vi "GUIAS CURVAS EM FUNÇÃO DO RAIO-3.vi"() -> ()   [LabVIEW 2014]
uses:
  <vilib>/Platform/TimedLoop/XDataNode/timing_clust.ctl
  <vilib>/Platform/TimedLoop/XDataNode/nitl_modes.ctl
  <vilib>/Platform/TimedLoop/XDataNode/wakeup.ctl
  <vilib>/Platform/TimedLoop/XDataNode/XDataNode.xnode
  <userlib>/Newport ESP301/Newport ESP301.lvlib
  <vilib>/Platform/TimedLoop/XDataNode/XDNodeRunTimeDep.lvlib
  <vilib>/Instr/_visa.llb/VISA Configure Serial Port (Instr).vi
panel:
  out "Raio":dbl
  out "PROGRESSÃO":i32
  in  "Raios":dbl[](array[numeric])=[100.0]
  in  "N_Guias":dbl=1.0
  in  "Iniciar":bool
  out "sin(x)":dbl
  in  "L":dbl=10.0 format="%.1f"
  in  "In.Curva":dbl=2.0
  out "Yin":dbl format="%.6g"
  out "Xin":dbl format="%.6g"
  out "d (um)":dbl
  in  "dist.":dbl=100.0
  in  "Stop Button":bool
  out "error out":errorcluster
  out "X (mm)":dbl format="%.2g"
  out "Y (um)":dbl format="%.1f"
  out "XY Graph":cluster{dbl[], dbl[]}(graph)={[0.0, 0.0, 0.0, 0.0, 0.0, 0.0, 0.0, 0.0, 0.0, 0.0, 0.0, 0.0, 0.0, 0.0, 0.0, 0.0, 0.0, 0.0, 0.0, 0.0, 0.0, 0.0, 0.0, 0.0, 0.0, 0.0, 0.0, 0.0, 0.0, 0.0, 0.0, 0.0, 0.0, 0.0, 0.0, 0.0, 0.0, 0.0, 0.0, 0.0, 0.0, 0.0, 0.0, 0.0, 0.0, 0.0, 0.0, 0.0, 0.0, 0.0, 0.0, 0.0, 0.0, 0.0, 0.0, 0.0, 0.0, 0.0, 0.0, 0.0, 0.0, 0.0, 0.0, 0.0, 0.0, 0.0, 0.0, 0.0, 0.0, 0.0, 0.0, 0.0, 0.0, 0.0, 0.0, 0.0], [4600.0, 4600.0, 4600.0, 4600.0, 4600.0, 4600.0, 4600.0, 4600.0, 4600.0, 4600.0, 4600.0, 4600.0, 4600.0, 4600.0, 4600.0, 4600.0, 4600.0, 4600.0, 4600.0, 4600.0, 4600.0, 4600.0, 4600.0, 4600.0, 4600.0, 4600.0, 4600.0, 4690.0, 4802.5, 4800.5, 4799.5, 4799.5, 4799.5, 4800.0, 4800.0, 4800.0, 4800.0, 4800.0, 4800.0, 4800.0, 4800.0, 4800.0, 4800.0, 4800.0, 4995.5, 5001.5, 5000.5, 5000.0, 5000.0, 4999.5, 4999.5, 5000.0, 5000.0, 5000.0, 5000.0, 5000.0, 5000.0, 5000.0, 5000.0, 5000.0, 5000.0, 5000.0, 5000.0, 5000.0, 5000.0, 5000.0, 5000.0, 5000.0, 5000.0, 5000.0, 5000.0, 5000.0, 5000.0, 5000.0, 5000.0, 5000.0]}
  in  "Refresh Button":bool
  in  "Velocity":dbl=3.0
  # "Inicio curva"
  # "Tamanho da amostra (mm)"
  # "Número guias curvas"
  # "Raio (mm)"
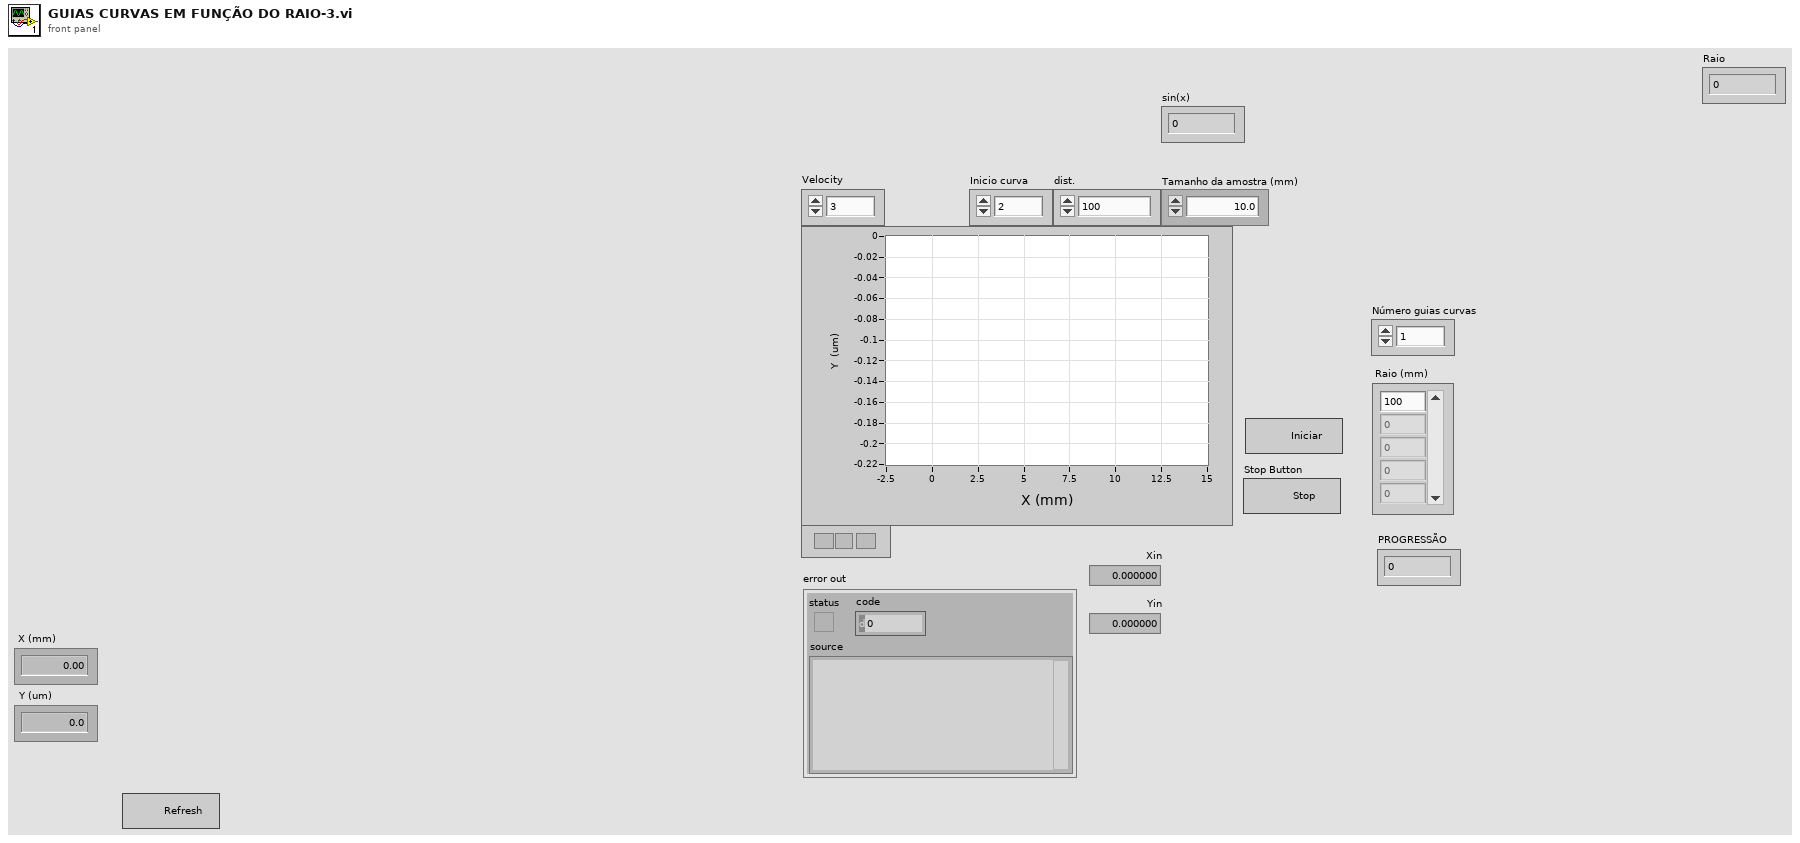
[diagram p1: front panel]
types:
  T1 = typedef "XDNodeRunTimeDep.lvlib/timing_clust.ctl" = cluster{"Expected End [f-1]":u64, "Actual End [f-1]":u64, "Finished Late? [f-1]":bool, "Expected End [i-1]":u64, "Actual End [i-1]":u64, "Finished Late? [i-1]":bool, "Expected Start [i]":u64, "Actual Start [i]":u64, "Expected Start [f]":u64, "Actual Start [f]":u64, "Source Name":string, "Structure Name":string, "Period":i64, "Deadline":i64, "Offset":i64, "Start":i64, "Priority":i32, "Timeout":i32, "Mode":T2, "Wakeup Reason":T3, "Error":errorcluster, "Source Type":string, "Secondary Source Type":string, "Global End Time":u64, "Global Start Time":u64, "Frame Duration":u64, "Iteration Duration":u64, "Assigned CPU":i32, "I/O Scan Engine Mode":u32}
  T2 = typedef "XDNodeRunTimeDep.lvlib/nitl_modes.ctl" = enum32{"No Change", "Process missed periods, maintain original phase", "Discard missed periods, maintain original phase", "Process missed periods, ignore original phase", "Discard missed periods, ignore original phase"}
  T3 = typedef "XDNodeRunTimeDep.lvlib/wakeup.ctl" = enum32{"Normal", "Aborted", "Asynchronous wakeup", "Timing source error", "Timed loop error", "Timeout"}
  T4 = cluster{"Axis1 moving":bool, "Axis2 moving":bool, "Axis3 moving":bool, "Axis4 moving":bool, "Motor Power of at least one axis":bool, "Reserved":bool, "Reserved":bool, "Reserved":bool, "Axis5 moving 2":bool, "Axis6 moving 2":bool, "Reserved":bool, "Reserved":bool, "Motor Power of at least one axis":bool, "Reserved":bool, "Reserved":bool, "Reserved":bool}
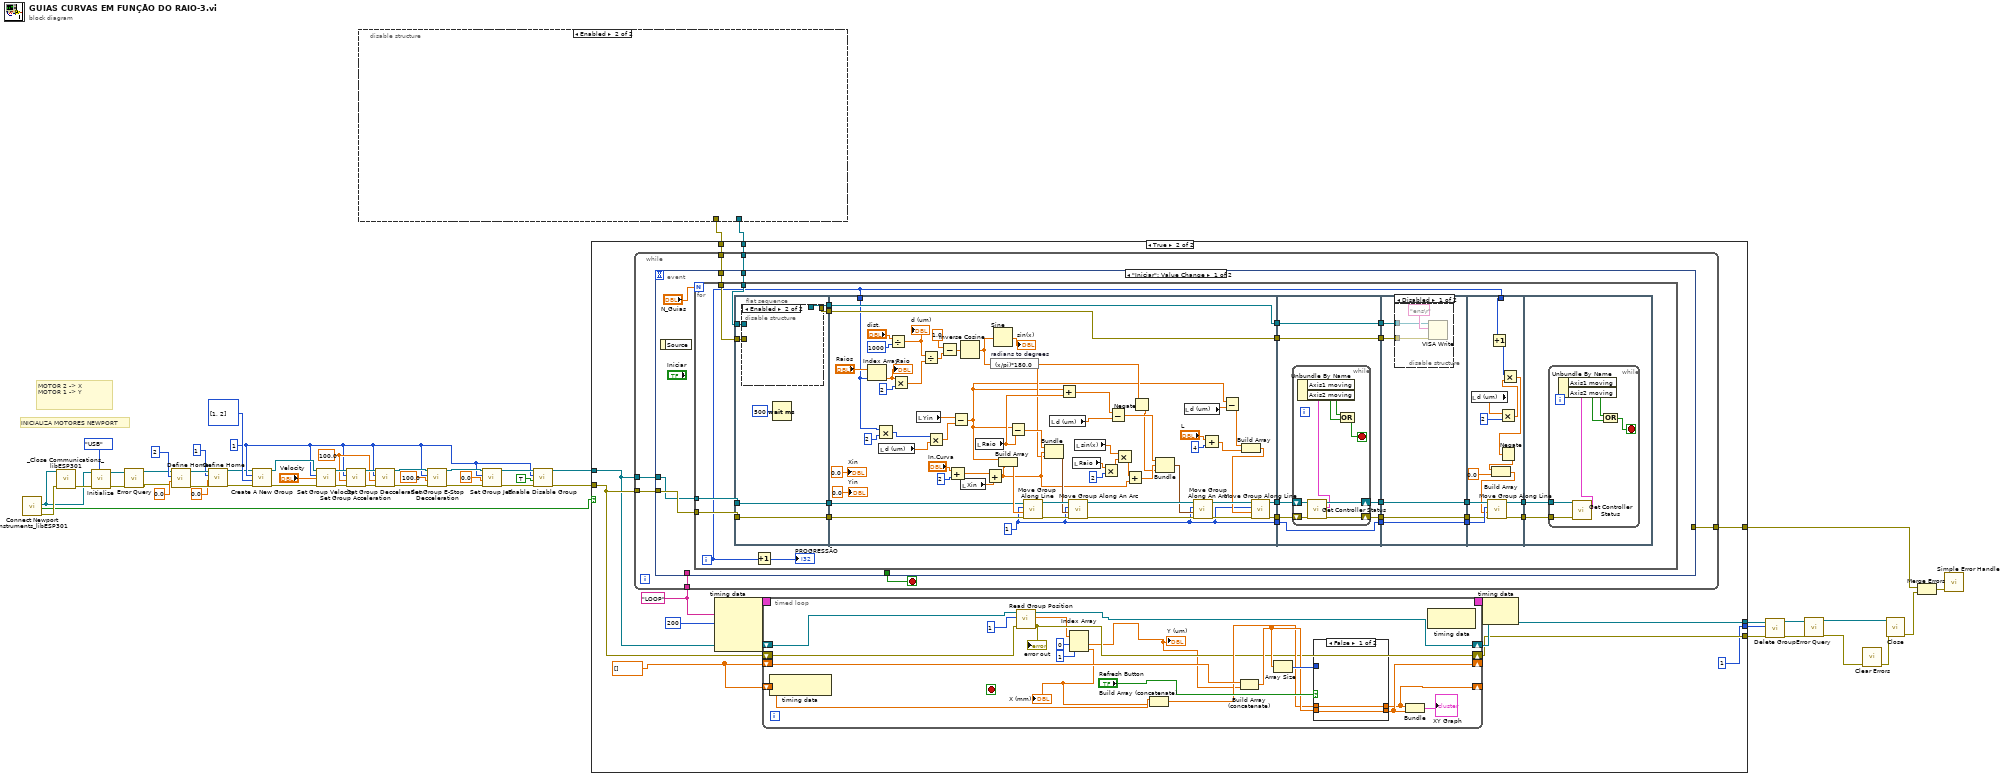
[diagram p0: block diagram]
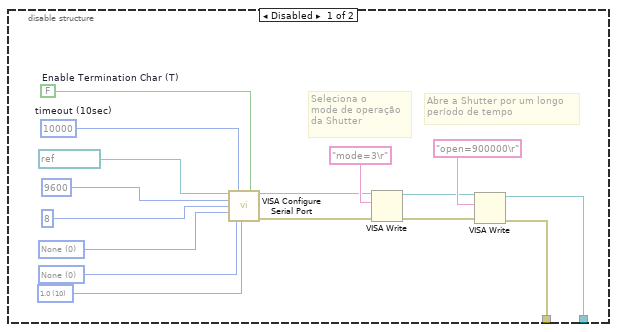
[diagram p2: hidden frame]
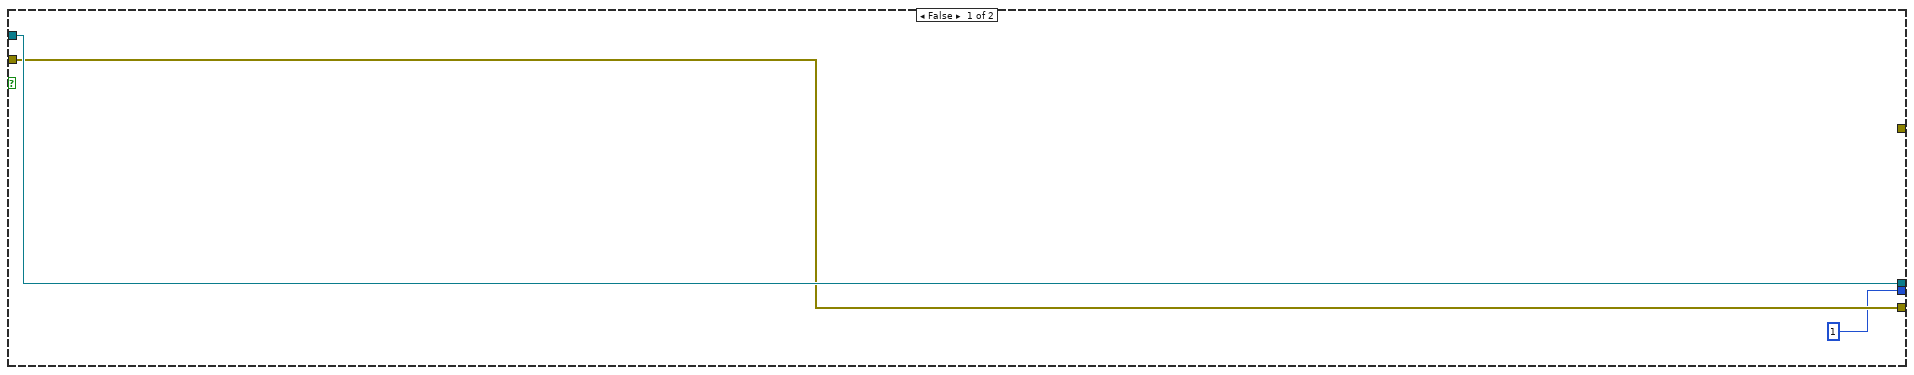
[diagram p3: hidden frame]
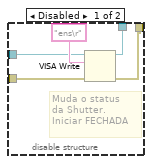
[diagram p4: hidden frame]
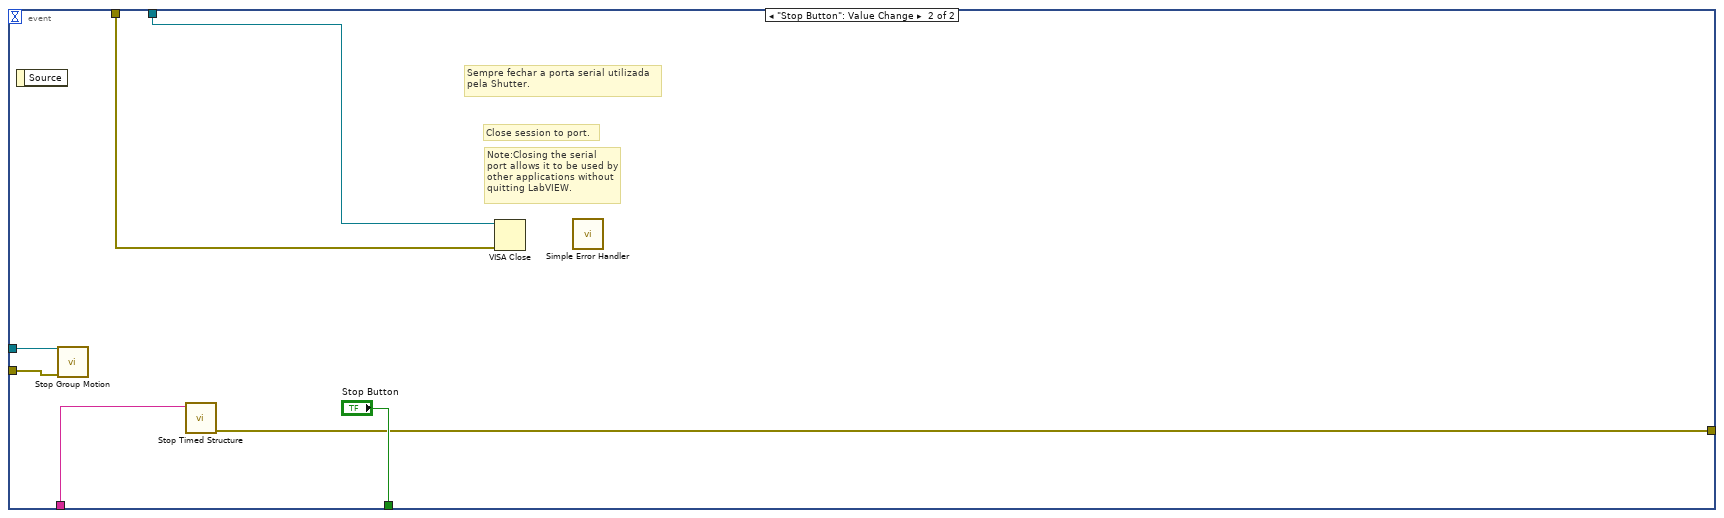
[diagram p6: hidden frame]
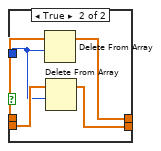
[diagram p7: hidden frame]
diagram:
  w21 = 1 ("Group #")
  w39 = 100.0 ("Acceleration (0 units/s²)")
  # "MOTOR 2 -> X\nMOTOR 1 -> Y"
  # "INICIALIZA MOTORES NEWPORT"
  n1 = call <userlib>:"Connect Newport Instruments_libESP301.vi"() -> ("error (duplicate)"=w49:errorcluster, "Connected"=w12:bool, "VISA resource name (duplicate)"=w48:refnum<visa-resource-name>)  [unwired: 7 in, 2 out]
  n2 = call <userlib>:"_Close Communications_libESP301.vi"("Instrument Channel"=w48, "error in (no error)"=w49) -> ("error out"=w51:errorcluster)  [unwired: 13 in]
  n3 = call <userlib>:"Initialize.vi"("VISA resource name"=w48, "error in (no error)"=w51, "Serial Link (RS232)"=enum16{"RS232", "USB"}."USB") -> ("VISA resource name out"=w29:refnum<visa-resource-name>, "error out"=w28:errorcluster)  [unwired: 6 in]
  n4 = call <userlib>:"Error Query.vi"("error in (no error)"=w28, "VISA resource name"=w29) -> ("error out"=w3:errorcluster, "VISA resource name out"=w4:refnum<visa-resource-name>)  [unwired: 2 in, 2 out]
  n5 = call <userlib>:"Define Home.vi"("error in (no error)"=w3, "Home Position (0 units)"=0.0, "Axis (1)"=2 ("y"), "VISA resource name"=w4) -> ("error out"=w9:errorcluster, "VISA resource name out"=w10:refnum<visa-resource-name>)  [unwired: 2 in]
  n6 = call <userlib>:"Define Home.vi"("error in (no error)"=w9, "Home Position (0 units)"=0.0, "Axis (1)"=1, "VISA resource name"=w10) -> ("error out"=w1:errorcluster, "VISA resource name out"=w2:refnum<visa-resource-name>)  [unwired: 2 in]
  n7 = call <userlib>:"Create A New Group.vi"("error in (no error)"=w1, "Axis Number"=i32[] [1, 2], "Group Number (1)"=w21, "VISA resource name"=w2) -> ("error out"=w45:errorcluster, "VISA resource name out"=w46:refnum<visa-resource-name>)  [unwired: 2 in]
  n8 = call <userlib>:"Set Group Velocity.vi"("error in (no error)"=w45, "Velocity (units/s)"="Velocity", "Group Number (1)"=w21, "VISA resource name"=w46) -> ("error out"=w40:errorcluster, "VISA resource name out"=w43:refnum<visa-resource-name>)  [unwired: 2 in]
  n9 = call <userlib>:"Set Group Acceleration.vi"("error in (no error)"=w40, "Acceleration (0 units/s²)"=w39, "Group Number (1)"=w21, "VISA resource name"=w43) -> ("error out"=w41:errorcluster, "VISA resource name out"=w42:refnum<visa-resource-name>)  [unwired: 2 in]
  n10 = disable-structure shown="Enabled" {
    disable-tunnel: [w53 _] -> w13
    disable-tunnel: [w52 _] -> w11
    frame Disabled {
      w62 = u16 0 items=["None", "Odd", "Even", "Mark", "Space"] ("parity")
      w65 = u16 10 items=["1.0"=10, "1.5"=15, "2.0"=20] ("stop bits")
      w66 = u16 0 items=["None"=0, "XON/XOFF"=1, "RTS/CTS"=2, "DTR/DSR"=4] ("flow control")
      w64 = FALSE  # Enable Termination Char (T)
      w63 = u32 10000  # timeout (10sec)
      # "Abre a Shutter por um longo\nperíodo de tempo"
      # "Seleciona o \nmode de operação\nda Shutter"
      n11 = call-poly "VISA Configure Serial Port"("VISA resource name"=refnum<visa-resource-name> "COM6", "timeout (10sec)"=w63, "Enable Termination\nChar (T)"=w64, "baud rate (9600)"=u32 9600 ("baud rate"), "data bits (8)"=u16 8 ("data bits"), "parity (0:none)"=w62, "stop bits (10: 1 bit)"=w65, "flow control (0:none)"=w66) -> ("VISA resource name out"=w58:refnum<visa-resource-name>, "error out"=w57:errorcluster)  [unwired: 6 in]
      n12 = VISA Write(VISA resource name=w58, write buffer="mode=3\r", error in (no error)=w57) -> (VISA resource name out=w55:refnum<visa-resource-name>, error out=w54:errorcluster)  [unwired: 1 out]
      n13 = VISA Write(VISA resource name=w55, write buffer="open=900000\r", error in (no error)=w54) -> (VISA resource name out=w53:refnum<visa-resource-name>, error out=w52:errorcluster)  [unwired: 1 out]
    }
    frame Enabled {
    }
  }
  n14 = call <userlib>:"Set Group Decceleration.vi"("error in (no error)"=w41, "Decceleration (0 units/s²)"=w39, "Group Number (1)"=w21, "VISA resource name"=w42) -> ("error out"=w35:errorcluster, "VISA resource name out"=w38:refnum<visa-resource-name>)  [unwired: 2 in]
  n15 = call <userlib>:"Set Group E-Stop Decceleration.vi"("error in (no error)"=w35, "E-Stop Decceleration (0 units/s²)"=100.0, "Group Number (1)"=w21, "VISA resource name"=w38) -> ("error out"=w34:errorcluster, "VISA resource name out"=w37:refnum<visa-resource-name>)  [unwired: 2 in]
  n16 = call <userlib>:"Set Group Jerk.vi"("error in (no error)"=w34, "Vector Jerk (0 units/s^3)"=0.0, "Group Number (1)"=w21, "VISA resource name"=w37) -> ("error out"=w33:errorcluster, "VISA resource name out"=w36:refnum<visa-resource-name>)  [unwired: 2 in]
  n17 = call <userlib>:"Enable Disable Group.vi"("error in (no error)"=w33, "Action (OFF)"=TRUE, "Group Number (1)"=w21, "VISA resource name"=w36) -> ("error out"=w22:errorcluster, "VISA resource name out"=w23:refnum<visa-resource-name>)  [unwired: 2 in]
  n18 = case shown="True" w12 {
    tunnel: [w70 w79] -> w27
    tunnel: [w69 w78] -> w26
    tunnel: [1 1] -> w25
    tunnel: w23 -> [w70 w75]
    tunnel: w22 -> [w69 w76]
    tunnel: [_ w73] -> w16
    tunnel: w13 -> [_ w72]
    tunnel: w11 -> [_ w71]
    frame False {
    }
    frame True {
      w80 = dbl[] []
      w74 = "LOOP" ("Structure Name")
      n19 = while {
        tunnel: w76 -> [w90]
        tunnel: w75 -> [w89]
        tunnel: w74 -> [w87]
        tunnel: [w86] -> w73
        tunnel: w72 -> [w85]
        tunnel: w71 -> [w84]
        stop <- w88 stop-if-true
        n20 = event shown="[0] \"Iniciar\": Value Change" {
          selector: _ -> [_ _]
          dyn-events: _ -> [_ _]
          timeout: _ -> [_ _]
          tunnel: w90 -> [w95 w240]
          tunnel: w89 -> [w94 w241]
          tunnel: [_ "Stop Button"] -> w88
          tunnel: w87 -> [_ w244]
          tunnel: [_ w243] -> w86
          tunnel: w85 -> [w92 w242]
          tunnel: w84 -> [w91 w239]
          event "Iniciar": Value Change {
            n21 = event-data() -> ()  [unwired: 1 in, 1 out]
            n22 = for {
              N: "N_Guias" -> [_]
              tunnel: w95 -> [w118]
              tunnel: w94 -> [w117]
              tunnel: w92 -> [w115]
              tunnel: w91 -> [w97]
              i -> [w96]
              n23 = flat-sequence {
                tunnel: w117 -> [w122]
                tunnel: w118 -> [w121]
                tunnel: [w121] -> w120
                tunnel: [w122] -> w119
                tunnel: w115 -> [w126]
                tunnel: [w125] -> w105
                tunnel: [w124] -> w102
                tunnel: w97 -> [w123]
                tunnel: w120 -> [w151]
                tunnel: w119 -> [w150]
                tunnel: w96 -> [w135]
                tunnel: [w144] -> w112
                tunnel: [w143] -> w111
                tunnel: [w142] -> w108
                tunnel: w105 -> [w140]
                tunnel: [w141] -> w103
                tunnel: w102 -> [w141]
                tunnel: [w140] -> w101
                tunnel: [w200] -> w113
                tunnel: w112 -> [w200]
                tunnel: w111 -> [w196]
                tunnel: [w194] -> w110
                tunnel: w108 -> [w197]
                tunnel: [w195] -> w107
                tunnel: [w199] -> w104
                tunnel: w103 -> [w199]
                tunnel: w101 -> [w198]
                tunnel: [w198] -> w100
                tunnel: [w213] -> w114
                tunnel: w113 -> [w213]
                tunnel: w110 -> [w212]
                tunnel: [w212] -> w109
                tunnel: w107 -> [w211]
                tunnel: [w211] -> w106
                tunnel: w104 -> [w210]
                tunnel: w100 -> [w209]
                tunnel: w114 -> [w230]
                tunnel: w109 -> [w229]
                tunnel: w106 -> [w228]
                tunnel: [w222] -> w99
                tunnel: [w221] -> w98
                tunnel: w96 -> [w220]
                tunnel: w99 -> [w232]
                tunnel: w98 -> [w231]
                frame #0 {
                  n24 = disable-structure shown="Enabled" {
                    disable-tunnel: w126 -> [w131 _]
                    disable-tunnel: [w130 _] -> w125
                    disable-tunnel: [w129 _] -> w124
                    disable-tunnel: w123 -> [w128 _]
                    frame Disabled {
                      # "Muda o status\nda Shutter.\nIniciar FECHADA"
                      n25 = VISA Write(VISA resource name=w131, write buffer="ens\r", error in (no error)=w128) -> (VISA resource name out=w130:refnum<visa-resource-name>, error out=w129:errorcluster)  [unwired: 1 out]
                    }
                    frame Enabled {
                    }
                  }
                  n26 = Wait (ms)(milliseconds to wait=u32 500) -> ()  [unwired: 1 out]
                }
                frame #1 {
                  w144 = 1 ("y")
                  n27 = Index Array(array="Raios", index=w135) -> (element=w145:dbl)
                  "Raio" <- w145
                  n28 = Multiply(x=w135, y=2) -> (x*y=w134:i32)
                  n29 = local read "d (um)"() -> (w133:dbl)
                  n30 = Divide(x="dist.", y=1000) -> (x/y=w183:dbl)
                  "d (um)" <- w183
                  n31 = Multiply(x=w145, y=2) -> (x*y=w189:dbl)
                  n32 = local read "Yin"() -> (w139:dbl)
                  n33 = Divide(x=w183, y=w189) -> (x/y=w186:dbl)
                  n34 = Multiply(x=w134, y=w133) -> (x*y=w138:dbl)
                  n35 = Subtract(x=1.0, y=w186) -> (x-y=w184:dbl)
                  n36 = Add(x="In.Curva", y=2) -> (x+y=w170:dbl)
                  n37 = Subtract(x=w139, y=w138) -> (x-y=w137:dbl)
                  n38 = Inverse Cosine(1:w184) -> (0:w172:dbl)
                  n39 = local read "Xin"() -> (w174:dbl)
                  n40 = local read "Raio"() -> (w162:dbl)
                  n41 = Add(x=w170, y=w174) -> (x+y=w164:dbl)
                  n42 = expression code="(x/pi)*180.0" "radians to degrees"(w172) -> (w153:dbl)
                  n43 = Sine(x=w172) -> (sin(x)=→"sin(x)":dbl)
                  n44 = Build Array(w137, w164) -> (w180:dbl[])
                  n45 = Subtract(x=w137, y=w162) -> (x-y=w173:dbl)
                  n46 = call <userlib>:"Move Group Along Line.vi"("error in (no error)"=w151, "Position (0 units)"=w180, "Group Number (1)"=w144, "VISA resource name"=w150) -> ("error out"=w178:errorcluster, "VISA resource name out"=w179:refnum<visa-resource-name>)  [unwired: 2 in]
                  n47 = Bundle(w173, w164, w153) -> (w177:cluster{dbl, dbl, dbl})  [unwired: 1 in]
                  n48 = local read "d (um)"() -> (w160:dbl)
                  n49 = Add(x=w137, y=w162) -> (x+y=w161:dbl)
                  n50 = call <userlib>:"Move Group Along An Arc.vi"("error in (no error)"=w178, "Arc  Parameters"=w177, "Group Number (1)"=w144, "VISA resource name"=w179) -> ("error out"=w192:errorcluster, "VISA resource name out"=w193:refnum<visa-resource-name>)  [unwired: 2 in]
                  n51 = local read "Raio"() -> (w168:dbl)
                  n52 = local read "sin(x)"() -> (w167:dbl)
                  n53 = Multiply(x=w168, y=2) -> (x*y=w166:dbl)
                  n54 = Subtract(x=w161, y=w160) -> (x-y=w159:dbl)
                  n55 = Multiply(x=w167, y=w166) -> (x*y=w165:dbl)
                  n56 = Add(x=w165, y=w164) -> (x+y=w163:dbl)
                  n57 = Negate(x=w153) -> (-x=w152:dbl)
                  n58 = Bundle(w159, w163, w152) -> (w191:cluster{dbl, dbl, dbl})  [unwired: 1 in]
                  n59 = local read "d (um)"() -> (w156:dbl)
                  n60 = call <userlib>:"Move Group Along An Arc.vi"("error in (no error)"=w192, "Arc  Parameters"=w191, "Group Number (1)"=w144, "VISA resource name"=w193) -> ("error out"=w149:errorcluster, "VISA resource name out"=w158:refnum<visa-resource-name>)  [unwired: 2 in]
                  n61 = Add(x="L", y=4) -> (x+y=w157:dbl)
                  n62 = Subtract(x=w137, y=w156) -> (x-y=w155:dbl)
                  n63 = Build Array(w155, w157) -> (w154:dbl[])
                  n64 = call <userlib>:"Move Group Along Line.vi"("error in (no error)"=w149, "Position (0 units)"=w154, "Group Number (1)"=w144, "VISA resource name"=w158) -> ("error out"=w143:errorcluster, "VISA resource name out"=w142:refnum<visa-resource-name>)  [unwired: 2 in]
                  "Xin" <- 0.0 ("Xin")
                  "Yin" <- 0.0 ("Yin")
                }
                frame #2 {
                  n65 = while {
                    shift-right: [w206] -> w195
                    shift-left: w197 -> [w208]
                    shift-right: [w205] -> w194
                    shift-left: w196 -> [w207]
                    stop <- w201 stop-if-true
                    n66 = call <userlib>:"Get Controller Status.vi"("error in (no error)"=w207, "VISA resource name"=w208) -> ("error out"=w205:errorcluster, "Controller Status"=w204:T4, "VISA resource name out"=w206:refnum<visa-resource-name>)  [unwired: 2 in, 1 out]
                    n67 = Unbundle By Name(w204) -> ("Axis1 moving"=w203:bool, "Axis2 moving"=w202:bool)
                    n68 = Compound Arithmetic op=OR(w203, w202) -> (w201:bool)
                  }
                }
                frame #3 {
                  n69 = disable-structure shown="Disabled" {
                    disable-tunnel: w210 -> [w215 _]
                    disable-tunnel: w209 -> [w214 _]
                    frame Disabled {
                      n70 = VISA Write(VISA resource name=w214, write buffer="ens\r", error in (no error)=w215) -> ()  [unwired: 3 out]
                    }
                    frame Enabled {
                    }
                  }
                }
                frame #4 {
                  n71 = local read "d (um)"() -> (w225:dbl)
                  n72 = Increment(x=w220) -> (x+1=w217:i32)
                  n73 = Multiply(x=w225, y=2) -> (x*y=w219:dbl)
                  n74 = Multiply(x=w217, y=w219) -> (x*y=w218:dbl)
                  n75 = Negate(x=w218) -> (-x=w223:dbl)
                  n76 = Build Array(w223, 0.0 ("element")) -> (w227:dbl[])
                  n77 = call <userlib>:"Move Group Along Line.vi"("error in (no error)"=w229, "Position (0 units)"=w227, "Group Number (1)"=w230, "VISA resource name"=w228) -> ("error out"=w221:errorcluster, "VISA resource name out"=w222:refnum<visa-resource-name>)  [unwired: 2 in]
                }
                frame #5 {
                  n78 = while {
                    tunnel: w232 -> [w234]
                    tunnel: w231 -> [w233]
                    stop <- w235 stop-if-true
                    n79 = call <userlib>:"Get Controller Status.vi"("error in (no error)"=w233, "VISA resource name"=w234) -> ("Controller Status"=w238:T4)  [unwired: 2 in, 3 out]
                    n80 = Unbundle By Name(w238) -> ("Axis1 moving"=w237:bool, "Axis2 moving"=w236:bool)
                    n81 = Compound Arithmetic op=OR(w237, w236) -> (w235:bool)
                  }
                }
              }
              n82 = Increment(x=w96) -> (x+1=→"PROGRESSÃO":i32)
            }
          }
          event "Stop Button": Value Change {
            # "Sempre fechar a porta serial utilizada\npela Shutter."
            # "Note:Closing the serial port allows it to be used by other applications without\nquitting LabVIEW."
            # "Close session to port."
            n83 = event-data() -> ()  [unwired: 1 in, 1 out]
            n84 = call <userlib>:"Stop Group Motion.vi"("error in (no error)"=w240, "VISA resource name"=w241) -> ()  [unwired: 4 in, 2 out]
            n85 = call <vilib>:"Stop Timed Structure.vi"("name"=w244) -> ("error out"=w243:errorcluster)  [unwired: 10 in]
            n86 = VISA Close(VISA resource name=w242, error in (no error)=w239) -> ()  [unwired: 1 out]
            n87 = call <vilib>:"Simple Error Handler.vi"() -> ()  [unwired: 5 in, 5 out]
          }
        }
      }
      n88 = node-c288(w74, i64 200 ("Period")) -> (w83:T1)  [unwired: 2 in]
      n89 = timed-loop {
        timing: w83 -> [_]
        timing-out: [_] -> w82
        shift-right: [w252] -> w79
        shift-left: w75 -> [w254]
        shift-right: [w251] -> w78
        shift-left: w76 -> [w253]
        shift-right: [w257] -> _
        shift-left: w80 -> [w261]
        shift-right: [w256] -> _
        shift-left: w80 -> [w259]
        stop <- _ stop-if-true
        n90 = node-c288() -> ()  [unwired: 1 in, 1 out]
        n91 = call <userlib>:"Read Group Position.vi"("error in (no error)"=w253, "Group Number (1)"=1, "VISA resource name"=w254) -> ("error out"=w251:errorcluster, "Position (units)"=w248:dbl[], "VISA resource name out"=w252:refnum<visa-resource-name>)  [unwired: 2 in]
        "error out" <- w251
        n92 = Index Array(array=w248, index #1=0 ("index"), index #2=1 ("index")) -> (element #1=w247:dbl, element #2=w246:dbl)
        "X (mm)" <- w246
        "Y (um)" <- w247
        n93 = Build Array (concatenate)(w259, w246) -> (w258:dbl[])
        n94 = Build Array (concatenate)(w261, w247) -> (w260:dbl[])
        n95 = Array Size(array=w260) -> (size(s)=w262:i32)
        n96 = case shown="False" "Refresh Button" {
          tunnel: [w266 w268] -> w256
          tunnel: w258 -> [w266 w271]
          tunnel: [w265 w267] -> w257
          tunnel: w260 -> [w265 w270]
          tunnel: w262 -> [_ w269]
          frame False {
          }
          frame True {
            n97 = Delete From Array(array=w271, length=w269) -> (array with subset deleted=w268:dbl[])  [unwired: 1 in, 1 out]
            n98 = Delete From Array(array=w270, length=w269) -> (array with subset deleted=w267:dbl[])  [unwired: 1 in, 1 out]
          }
        }
        n99 = Bundle(w256, w257) -> (→"XY Graph":cluster{dbl[], dbl[]})  [unwired: 1 in]
        n100 = node-c288() -> ()  [unwired: 1 in, 1 out]
      }
      n101 = node-c288(w82) -> ()  [unwired: 1 out]
    }
  }
  n102 = call <userlib>:"Delete Group.vi"("error in (no error)"=w26, "Group Number (1)"=w25, "VISA resource name"=w27) -> ("error out"=w19:errorcluster, "VISA resource name out"=w20:refnum<visa-resource-name>)  [unwired: 3 in]
  n103 = call <userlib>:"Error Query.vi"("error in (no error)"=w19, "VISA resource name"=w20) -> ("error out"=w17:errorcluster, "VISA resource name out"=w18:refnum<visa-resource-name>)  [unwired: 2 in, 2 out]
  n104 = call <vilib>:"Clear Errors.vi"("error in (no error)"=w17) -> ("error out"=w24:errorcluster)  [unwired: 5 in, 1 out]
  n105 = call <userlib>:"Close.vi"("error in (no error)"=w24, "VISA resource name"=w18) -> ("error out"=w15:errorcluster)  [unwired: 9 in]
  n106 = Merge Errors(w16, w15) -> (w14:errorcluster)
  n107 = call <vilib>:"Simple Error Handler.vi"("error in (no error)"=w14) -> ()  [unwired: 4 in, 5 out]
